vi "Get_Temp_and_Press.vi"(4 "Averaging time (mins)":dbl=5.0 format="%.2f") -> (0 "Abs Press (mbar)":dbl format="%.2f", 2 "Temperature":dbl format="%.2f")   [LabVIEW 2012]
uses:
  Controls/Server_Comms.ctl
  ADAM Client/Sub VIs/ADAM Controls/Module_type_ADAM.ctl
  ADAM Client/Sub VIs/ADAM Controls/Calib_type_ADAM.ctl
  Controls/Global_mode.ctl
  ADAM Client/Sub VIs/ADAM Controls/Ch_description_ADAM.ctl
  ADAM Client/Sub VIs/ADAM Controls/Function_ADAM.ctl
  ADAM Client/Sub VIs/ADAM Controls/Channel_State.ctl
  ADAM Client/Sub VIs/ADAM Controls/Address.ctl
  ADAM Client/Sub VIs/ADAM Controls/Update_scan_value.ctl
  Globals/Preference_global.vi
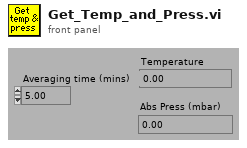
[diagram p1: front panel]
types:
  T1 = typedef "Server_Comms.ctl" = enum16{"Server Link Healthy", "Do Not Link To Server"}
  T2 = typedef "Update_scan_value.ctl" = cluster{"Channel Name":string, "New Value":dbl}
  T3 = typedef "Ch_description_ADAM.ctl" = cluster{"Ch Name":string, "Type":T4, "Function":T5, "Ch State":T6, "Calibration type":T7, "A":dbl, "B":dbl, "C":dbl, "D":dbl, "Comments":string, "Address":T8, "String":string, "Duty":u16}
  T4 = typedef "Module_type_ADAM.ctl" = string
  T5 = typedef "Function_ADAM.ctl" = enum16{"Analogue Input", "Digital Input", "Event counter", "Event rate", "Analogue Output", "Digital Output", "Relay Output"}
  T6 = typedef "Channel_State.ctl" = enum16{"On", "Off", "Always On", "Always Off"}
  T7 = typedef "Calib_type_ADAM.ctl" = enum16{"Raw", "Bx + A", "Cx^2 + Bx + A", "Dx^3 + Cx^2 + Bx + A", "In Band", "Hi-Tec Q", "Hi-Tec M_dot", "Text"}
  T8 = typedef "Address.ctl" = cluster{"Main":i32, "Ch.":i32, "Sub":i32, "Port Name":string}
  T9 = typedef "Global_mode.ctl" = enum16{"Read Global", "Load Global From File", "Write Global to File"}
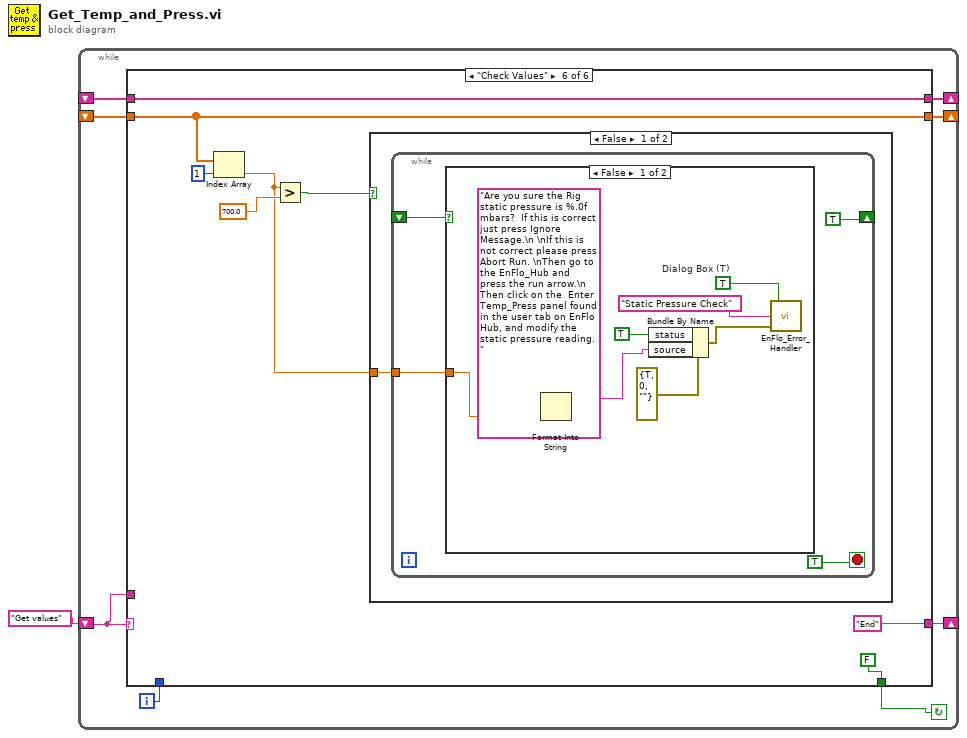
[diagram p0: block diagram]
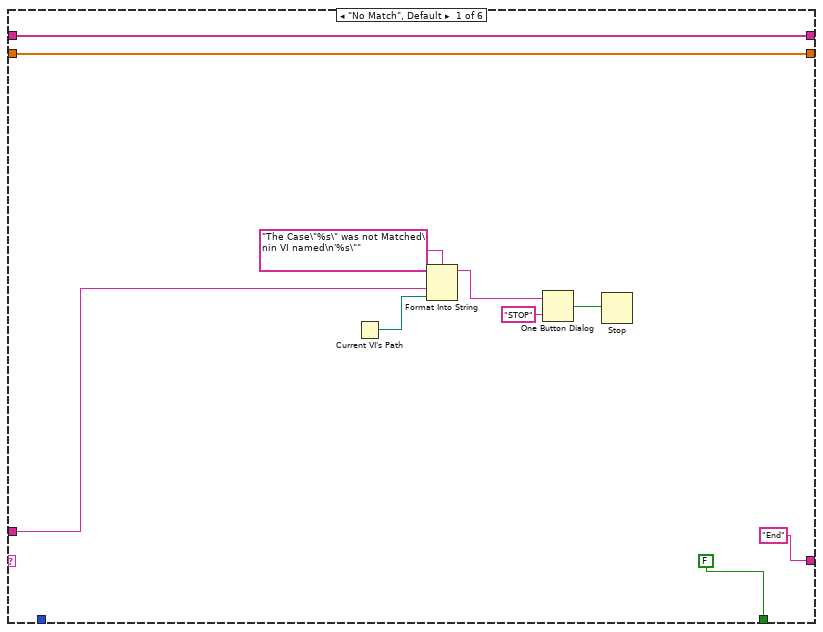
[diagram p2: hidden frame]
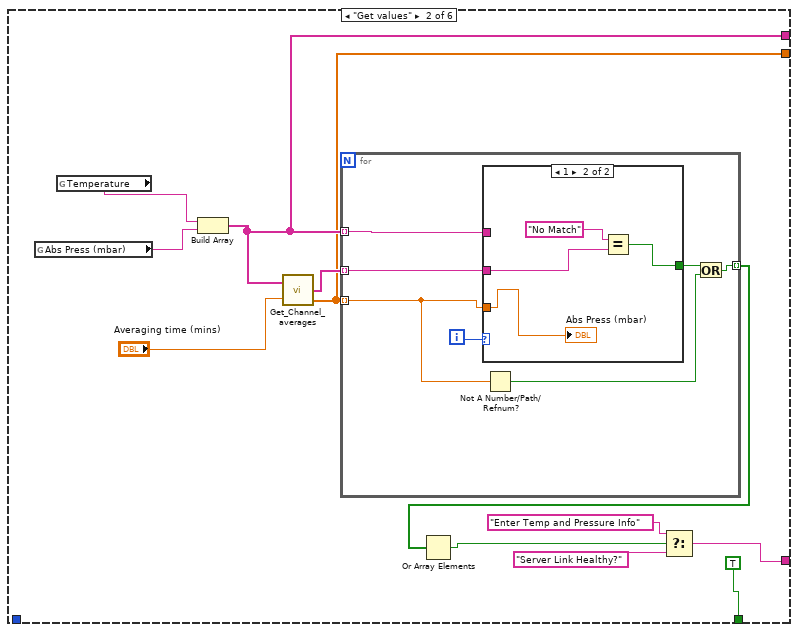
[diagram p3: hidden frame]
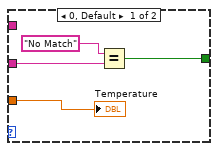
[diagram p4: hidden frame]
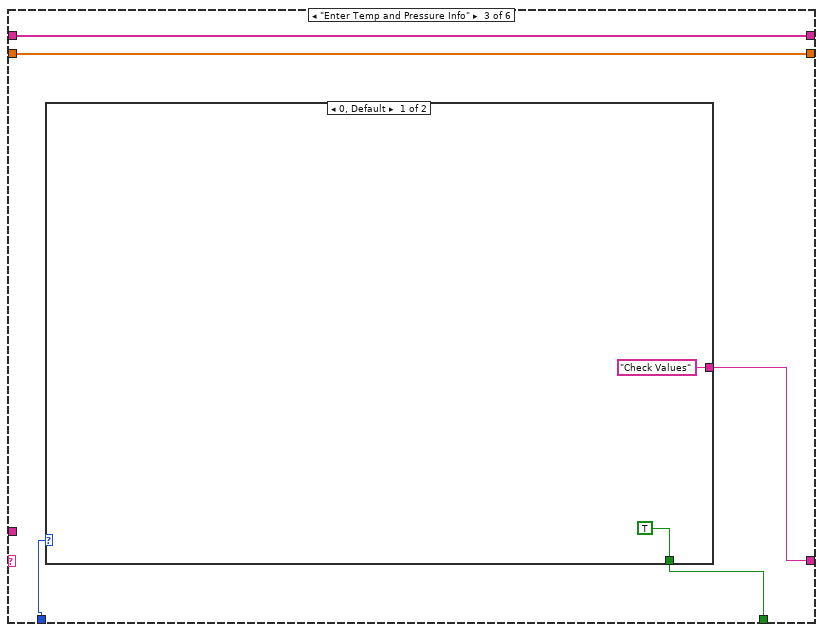
[diagram p5: hidden frame]
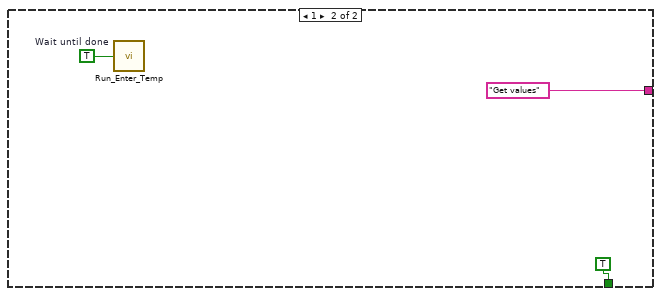
[diagram p6: hidden frame]
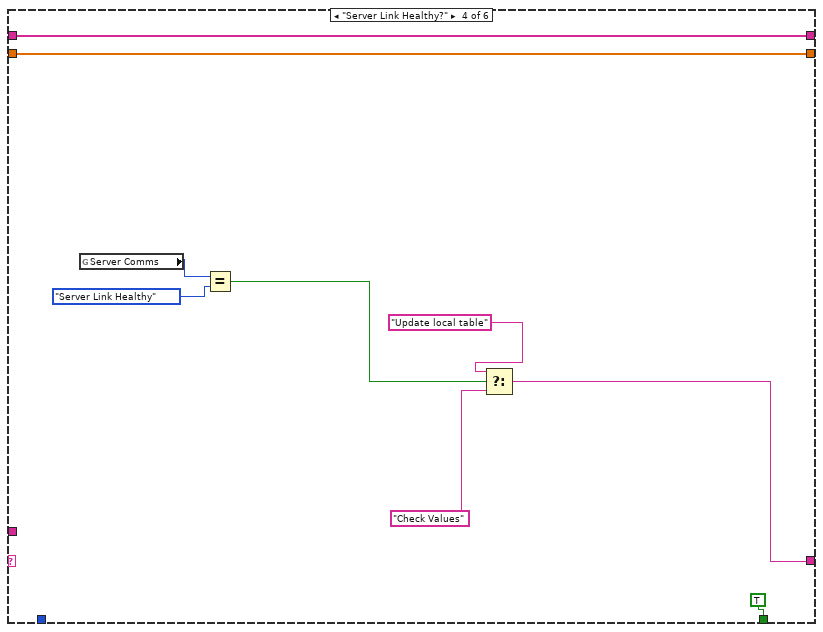
[diagram p7: hidden frame]
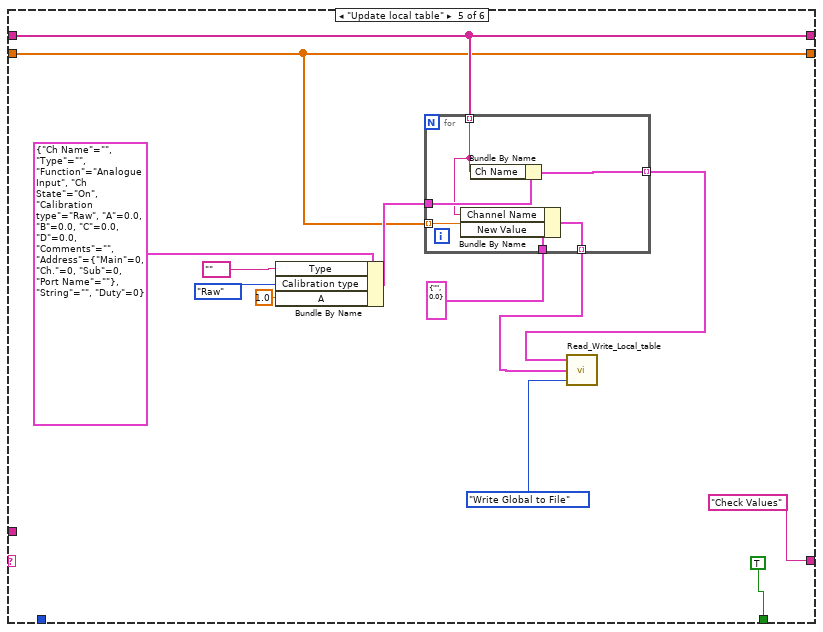
[diagram p8: hidden frame]
diagram:
  n1 = while {
    shift-right: [w8] -> _
    shift-left: "Get values" -> [w7]
    shift-right: [w6] -> _
    shift-left: _ -> [w4]
    shift-right: [w5] -> _
    shift-left: _ -> [w3]
    i -> [w2]
    stop <- w9 continue-if-true
    n2 = case shown="\"Check Values\"" w7 {
      tunnel: [FALSE TRUE w47 TRUE TRUE FALSE] -> w9
      tunnel: ["End" w25 w49 w59 "Check Values" "End"] -> w8
      tunnel: w7 -> [w14 _ _ _ _ _]
      tunnel: [w11 w22 w51 w65 w69 w90] -> w6
      tunnel: [w10 w20 w50 w64 w67 w89] -> w5
      tunnel: w4 -> [w11 _ w51 w65 w69 w90]
      tunnel: w3 -> [w10 _ w50 w64 w67 w89]
      tunnel: w2 -> [_ _ w48 _ _ _]
      frame "No Match", Default {
        n3 = Current VI's Path() -> (path=w19:path)
        n4 = Format Into String(format string="The Case\"%s\" was not Matched\nin VI named\n'%s\"" ("Format String"), w14, w19) -> (resulting string=w16:string)  [unwired: 2 in, 1 out]
        n5 = One Button Dialog(message=w16, button name ("OK")="STOP") -> (true=w18:bool)
        n6 = Stop(stop? (T)=w18) -> ()
      }
      frame "Get values" {
        n7 = global read "Preference_global.vi" "Abs Press (mbar)"() -> (w31:string)
        n8 = global read "Preference_global.vi" "Temperature"() -> (w30:string)
        n9 = Build Array(w30, w31) -> (w22:string[])
        n10 = call "Get_Channel_averages.vi"("Desired Ch Names"=w22, "Averaging time (mins)"="Averaging time (mins)") -> ("Values"=w21:string[], "number"=w20:dbl[])  [unwired: 1 in, 1 out]
        n11 = for {
          tunnel: w22 -> [w37] mode=indexing
          tunnel: w20 -> [w35] mode=indexing
          tunnel: w21 -> [w36] mode=indexing
          tunnel: [w34] -> w27 mode=indexing
          i -> [w38]
          n12 = case shown="1" w38 {
            tunnel: w35 -> [w42 w43]
            tunnel: w37 -> [_ _]
            tunnel: w36 -> [w40 w45]
            tunnel: [w39 w44] -> w33
            frame 0, Default {
              n13 = Equal?(x="No Match", y=w40) -> (x = y?=w39:bool)
              "Temperature" <- w42
            }
            frame 1 {
              n14 = Equal?(x="No Match", y=w45) -> (x = y?=w44:bool)
              "Abs Press (mbar)" <- w43
            }
          }
          n15 = Not A Number/Path/Refnum?(number/path/refnum=w35) -> (NaN/Path/Refnum?=w32:bool)
          n16 = Or(x=w33, y=w32) -> (x .or. y?=w34:bool)
        }
        n17 = Or Array Elements(Boolean array=w27) -> (logical OR=w26:bool)
        n18 = Select(t="Enter Temp and Pressure Info", s=w26, f="Server Link Healthy?") -> (s? t:f=w25:string)
      }
      frame "Enter Temp and Pressure Info" {
        n19 = case shown="0, Default" w48 {
          tunnel: ["Check Values" "Get values"] -> w49
          tunnel: [TRUE TRUE] -> w47
          frame 0, Default {
          }
          frame 1 {
            w54 = TRUE  # Wait until done
            n20 = call "Run_Enter_Temp.vi"("Wait until done"=w54) -> ()  [unwired: 1 out]
          }
        }
      }
      frame "Server Link Healthy?" {
        n21 = global read "Preference_global.vi" "Server Comms"() -> (w62:T1)
        n22 = Equal?(x=w62, y=Server_Comms."Server Link Healthy" ("Server Comms")) -> (x = y?=w61:bool)
        n23 = Select(t="Update local table", s=w61, f="Check Values") -> (s? t:f=w59:string)
      }
      frame "Update local table" {
        n24 = Bundle By Name(cluster=T3 {"Ch Name"="", "Type"="", "Function"=enum."Analogue Input", "Ch State"=enum."On", "Calibration type"=enum."Raw", "A"=0.0, "B"=0.0, "C"=0.0, "D"=0.0, "Comments"="", "Address"={"Main"=0, "Ch."=0, "Sub"=0, "Port Name"=""}, "String"="", "Duty"=0} ("Ch Discription"), "Type"=T4 "", "Calibration type"=Calib_type_ADAM."Raw", "A"=1.0) -> (w72:T3)
        n25 = for {
          tunnel: w72 -> [w84]
          tunnel: [w83] -> w70 mode=indexing
          tunnel: w69 -> [w81] mode=indexing
          tunnel: T2 {"Channel Name"="", "New Value"=0.0} ("Update Scan Value Cluster") -> [w82]
          tunnel: w67 -> [w80] mode=indexing
          tunnel: [w79] -> w66 mode=indexing
          n26 = Bundle By Name(cluster=w82, "Channel Name"=w81, "New Value"=w80) -> (w79:T2)
          n27 = Bundle By Name(cluster=w84, "Ch Name"=w81) -> (w83:T3)
        }
        n28 = call "Read_Write_Local_table.vi"("Mode"=Global_mode."Write Global to File", "Ch Values in"=w66, "Channels Descriptions In"=w70) -> ()  [unwired: 3 out]
      }
      frame "Check Values" {
        n29 = Index Array(array=w89, index=1) -> (element=w85:dbl)
        n30 = Greater?(x=w85, y=700.0) -> (0:w86:bool)
        n31 = case shown="False" w86 {
          tunnel: w85 -> [w93 _]
          frame False {
            n32 = while {
              shift-right: [TRUE] -> _
              shift-left: _ -> [w96]
              tunnel: w93 -> [w95]
              stop <- TRUE stop-if-true
              n33 = case shown="False" w96 {
                tunnel: w95 -> [w100 _]
                frame False {
                  w101 = TRUE  # Dialog Box (T)
                  n34 = Format Into String(format string="Are you sure the Rig static pressure is %.0f mbars?  If this is correct just press Ignore Message.\n \nIf this is not correct please press Abort Run. \nThen go to the EnFlo_Hub and press the run arrow.\n Then click on the  Enter Temp_Press panel found in the user tab on EnFlo Hub, and modify the static pressure reading.", w100) -> (resulting string=w98:string)  [unwired: 2 in, 1 out]
                  n35 = Bundle By Name(cluster=errorcluster {"status"=TRUE, "code"=0, "source"=""} ("error in (no error)"), "status"=TRUE, "source"=w98) -> (w104:errorcluster)
                  n36 = call "EnFlo_Error_Handler.vi"("error in (no error)"=w104, "Error Type"="Static Pressure Check", "Dialog Box (T)"=w101) -> ()  [unwired: 3 out]
                }
                frame True {
                }
              }
            }
          }
          frame True {
          }
        }
      }
    }
  }
